vi "Start.vi"(8 "error in (no error)":errorcluster, 11 "RIO_API in":refnum<class "9770 API.lvclass">) -> (0 "error out":errorcluster, 3 "RIO_API out":refnum<class "9770 API.lvclass">)   [LabVIEW 2017, in "9770 API.lvclass"]
uses:
  <vilib>/addons/InsightCM/Devices/Shared/Emsa/Emsa9770API/9770 API.lvclass
  <vilib>/addons/InsightCM/Devices/Shared/Emsa/Emsa9770API/9770 API.lvclass/9770 API.ctl
  <vilib>/Utility/error.llb/Error Cluster From Error Code.vi
  <vilib>/rvi/errors/niLvFpgaAdjustHostInterfaceError.vi
  <vilib>/rvi/interface/nirviReadWriteControl/nirviReadWriteControl.xnode
  <vilib>/addons/InsightCM/Devices/Shared/Emsa/Emsa9770API/controls/FPGATypeDef.ctl
  NiFpgaLv.dll
  <vilib>/rvi/interface/Simulation/niFpgaSimulationCallBeginRW.vi
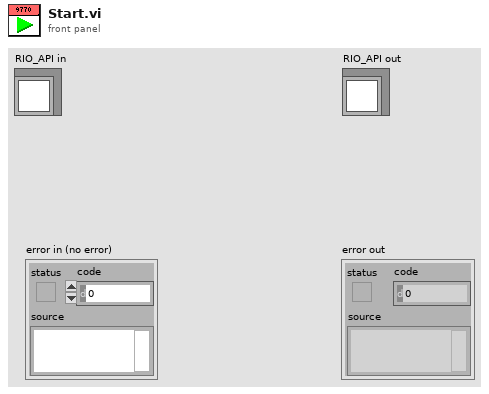
[diagram p1: front panel]
types:
  T1 = typedef "9770 API.lvclass/FPGATypeDef.ctl" = refnum<k20>
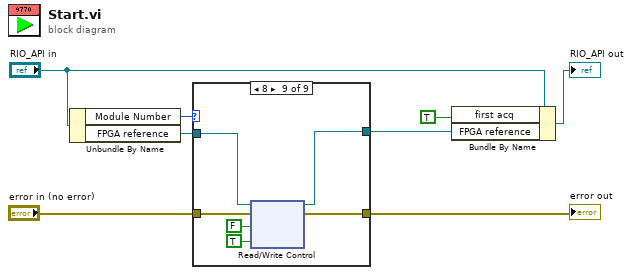
[diagram p0: block diagram]
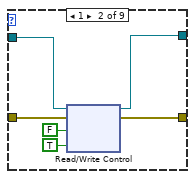
[diagram p3: hidden frame]
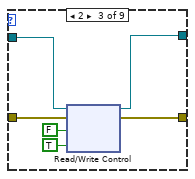
[diagram p4: hidden frame]
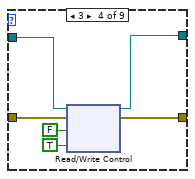
[diagram p5: hidden frame]
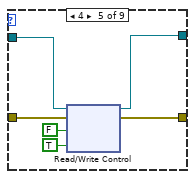
[diagram p6: hidden frame]
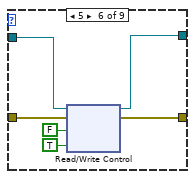
[diagram p7: hidden frame]
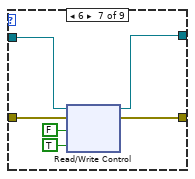
[diagram p8: hidden frame]
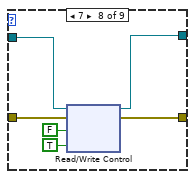
[diagram p9: hidden frame]
diagram:
  n1 = Unbundle By Name("RIO_API in") -> ("Module Number"=w3:u32, "FPGA reference"=w2:T1)
  n2 = case shown="8" w3 {
    tunnel: "error in (no error)" -> [w10 w16 w22 w28 w34 w40 w46 w52 w58]
    tunnel: [w10 w15 w21 w27 w33 w39 w45 w51 w57] -> w7
    tunnel: w2 -> [w9 w14 w20 w26 w32 w38 w44 w50 w56]
    tunnel: [w9 w13 w19 w25 w31 w37 w43 w49 w55] -> w1
    frame 0, Default {
    }
    frame 1 {
      n3 = xnode "Read/Write Control"("FPGA VI Reference In"=w14, "error in"=w16, "Stop 1"=FALSE ("Start 1"), "Start 1"=TRUE ("Stop 1")) -> ("FPGA VI Reference Out"=w13:T1, "error out"=w15:errorcluster)
    }
    frame 2 {
      n4 = xnode "Read/Write Control"("FPGA VI Reference In"=w20, "error in"=w22, "Stop 2"=FALSE ("Start 1"), "Start 2"=TRUE ("Stop 2")) -> ("FPGA VI Reference Out"=w19:T1, "error out"=w21:errorcluster)
    }
    frame 3 {
      n5 = xnode "Read/Write Control"("FPGA VI Reference In"=w26, "error in"=w28, "Stop 3"=FALSE ("Start 1"), "Start 3"=TRUE ("Stop 3")) -> ("FPGA VI Reference Out"=w25:T1, "error out"=w27:errorcluster)
    }
    frame 4 {
      n6 = xnode "Read/Write Control"("FPGA VI Reference In"=w32, "error in"=w34, "Stop 4"=FALSE ("Start 1"), "Start 4"=TRUE ("Stop 4")) -> ("FPGA VI Reference Out"=w31:T1, "error out"=w33:errorcluster)
    }
    frame 5 {
      n7 = xnode "Read/Write Control"("FPGA VI Reference In"=w38, "error in"=w40, "Stop 5"=FALSE ("Start 1"), "Start 5"=TRUE ("Stop 5")) -> ("FPGA VI Reference Out"=w37:T1, "error out"=w39:errorcluster)
    }
    frame 6 {
      n8 = xnode "Read/Write Control"("FPGA VI Reference In"=w44, "error in"=w46, "Stop 6"=FALSE ("Start 1"), "Start 6"=TRUE ("Stop 6")) -> ("FPGA VI Reference Out"=w43:T1, "error out"=w45:errorcluster)
    }
    frame 7 {
      n9 = xnode "Read/Write Control"("FPGA VI Reference In"=w50, "error in"=w52, "Stop 7"=FALSE ("Start 1"), "Start 7"=TRUE ("Stop 7")) -> ("FPGA VI Reference Out"=w49:T1, "error out"=w51:errorcluster)
    }
    frame 8 {
      n10 = xnode "Read/Write Control"("FPGA VI Reference In"=w56, "error in"=w58, "Stop 8"=FALSE ("Start 1"), "Start 8"=TRUE ("Stop 8")) -> ("FPGA VI Reference Out"=w55:T1, "error out"=w57:errorcluster)
    }
  }
  "error out" <- w7
  n11 = Bundle By Name(cluster="RIO_API in", "first acq"=TRUE, "FPGA reference"=w1) -> (→"RIO_API out":refnum<class "9770 API.lvclass">)
